vi "niScope Is Device Ready.vi"(8 "error in":errorcluster, 11 "resource name":refnum<k15>="DAQ::1") -> (0 "error out":errorcluster, 2 "Device Ready?":bool)   [LabVIEW 2011]
doc: "Returns whether the device is ready to be used to the <B>Device Ready?</B> parameter."
uses:
  niScope_32.dll
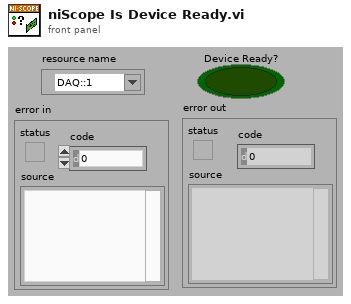
[diagram p1: front panel]
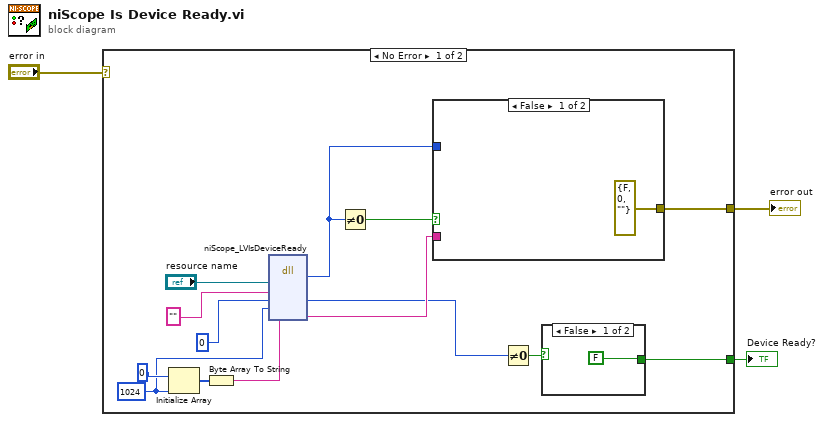
[diagram p0: block diagram]
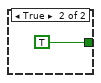
[diagram p2: hidden frame]
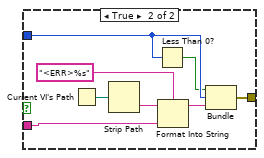
[diagram p3: hidden frame]
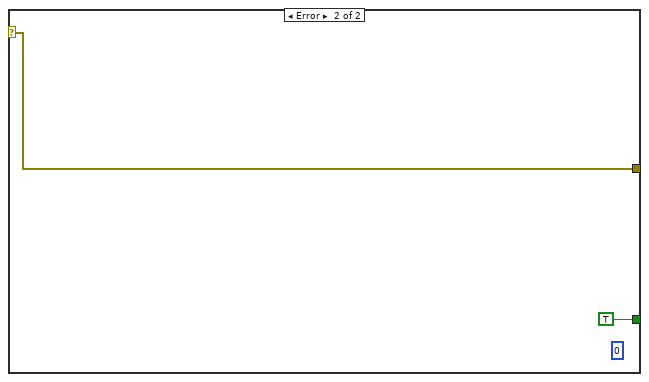
[diagram p4: hidden frame]
diagram:
  n1 = case shown="No Error" "error in" {
    selector: "error in" -> [_ w30]
    tunnel: [w8 w30] -> w2
    tunnel: [w5 TRUE] -> w1
    frame No Error {
      w13 = 1024
      n2 = Initialize Array(0, w13) -> (w15:i32[])
      n3 = Byte Array To String(unsigned byte array=w15) -> (string=w12:string)
      n4 = dll-call lib="niScope_*.*" fn="niScope_LVIsDeviceReady" ("niScope_*.*:niScope_LVGetDeviceStatus")("resourceName"="resource name", "channel"="", "deviceReady"=0 ("deviceStatus"), "errorBufferSize"=w13, "errorBuffer"=w12) -> ("status"=w10:i32, "deviceReady"=w6:u16, "errorBuffer"=w9:string)  [unwired: 6 in, 2 out]
      n5 = Not Equal To 0?(x=w10) -> (x != 0?=w11:bool)
      n6 = case shown="False" w11 {
        tunnel: w9 -> [_ w28]
        tunnel: w10 -> [_ w23]
        tunnel: [cluster{bool, "status":i32, string} {FALSE, "status"=0, ""} w21] -> w8
        frame False {
        }
        frame True {
          n7 = Current VI's Path() -> (path=w26:path)
          n8 = Strip Path(path=w26) -> (name=w25:string)  [unwired: 1 out]
          n9 = Less Than 0?(x=w23) -> (x < 0?=w22:bool)
          n10 = Format Into String(format string="<ERR>%s", initial string=w25, w28) -> (resulting string=w24:string)  [unwired: 1 in, 1 out]
          n11 = Bundle(w22, "status"=w23, w24) -> (w21:cluster{bool, "status":i32, string})  [unwired: 1 in]
        }
      }
      n12 = Not Equal To 0?(x=w6) -> (x != 0?=w7:bool)
      n13 = case shown="False" w7 {
        tunnel: [FALSE TRUE] -> w5
        frame False {
        }
        frame True {
        }
      }
    }
    frame Error {
      (unwired) 0 ("deviceStatus")
    }
  }
  "error out" <- w2
  "Device Ready?" <- w1
